vi "vision testing.vi"() -> ()   [LabVIEW 2013]
doc: "This VI demonstrates how to do target processing on a laptop computer. It uses the same MJPG VI as the dashboard, sets a few of the important camera properties that impact processing, and carries out the same processing steps as the RT example also included in this project."
uses:
  <vilib>/Rock Robotics/WPI/Camera/WPI_CameraImageSize.ctl
  <vilib>/vision/Image Controls.llb/IMAQ Image.ctl
  <vilib>/Rock Robotics/WPI/Camera/WPI_CameraWhite Balance Values.ctl
  <vilib>/Rock Robotics/WPI/Camera/WPI_CameraExposure Values.ctl
  <vilib>/Rock Robotics/WPI/Camera/WPI_CameraFrameRate.ctl
  <vilib>/vision/NI_Vision_Development_Module.lvlib
panel:
  out "final image":T1(plugin-control)
  in  "Pre-Process":bool
  out "mspi":u32=9
  in  "Numeric":i32=1
  out "y":dbl
  out "x":dbl
  out "Image Out":T1
  out "error out":errorcluster
  out "Number Found":i32
  in  "Camera Settings":T3={"FPS"=7, "Compression"=40, "Image Size"=enum."160x120"}
  in  "Camera IP Address":string="10.11.24.11"
  out "Original Image":T1(plugin-control)
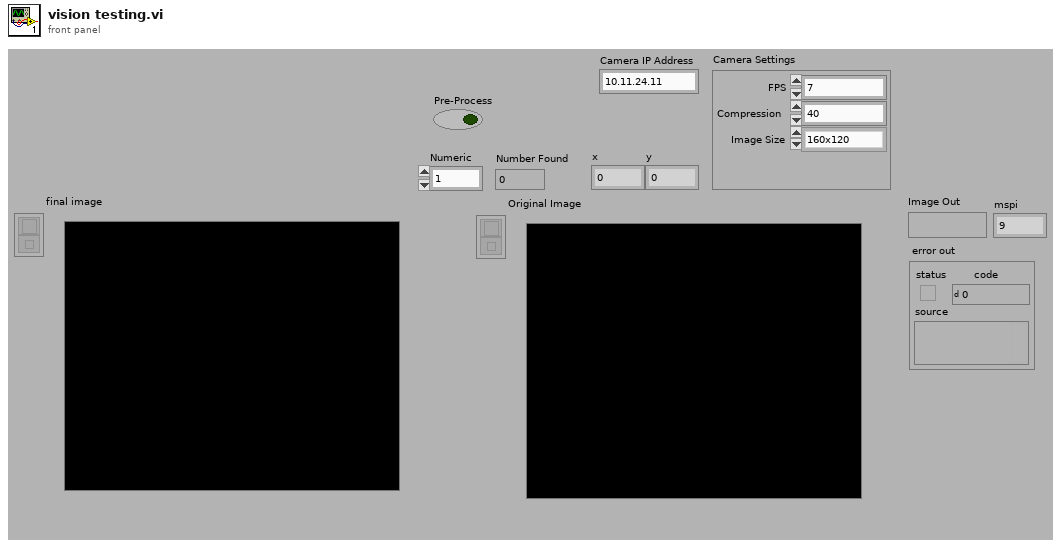
[diagram p1: front panel]
types:
  T1 = typedef "IMAQ Image.ctl" = refnum<image>
  T2 = typedef "WPI_CameraImageSize.ctl" = enum16{"640x480", "320x240", "160x120"}
  T3 = cluster{"FPS":i32, "Compression":i32, "Image Size":T2}
  T4 = typedef "Image Type" = u32
  T5 = typedef "WPI_CameraFrameRate.ctl" = u32
  T6 = typedef "WPI_CameraExposure Values.ctl" = enum16{"Auto", "Flicker-free 50 Hz", "Flicker-free 60 Hz", "Hold current"}
  T7 = typedef "WPI_CameraWhite Balance Values.ctl" = enum16{"Auto", "Fixed indoor", "Fixed outdoor 1", "Fixed outdoor 2", "Fixed fluorescent 1", "Fixed fluorescent 2", "Hold current"}
  T8 = typedef "WPI_CameraDevRef.ctl" = cluster{"Camera Address":string, "CameraStatus":errorcluster, "Acquire Image Notifier":refnum<notifier>}
  T9 = enum32{"AutoM", "Close", "Dilate", "Erode", "Gradient", "Gradient out", "Gradient in", "Hit miss", "Open", "PClose", "POpen", "Thick", "Thin"}
  T10 = cluster{"Brightness":sgl, "Contrast":sgl, "Gamma":sgl}
  T11 = cluster{"Measurement Parameter":i32, "Range Lower Value":dbl, "Range Upper Value":dbl, "Range":bool, "Measurement Type":bool}[]
  T12 = typedef "Particle Parameters" = i32
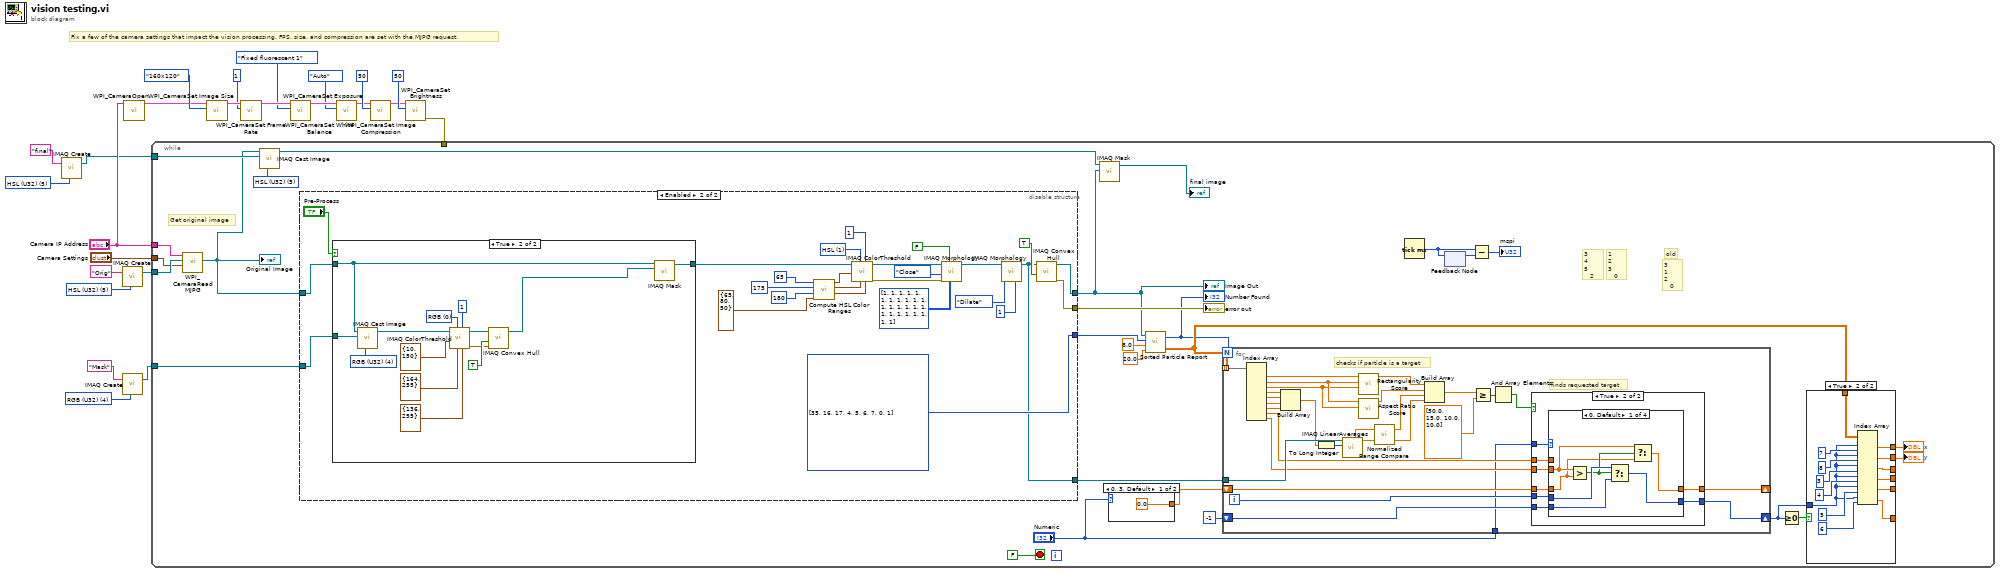
[diagram p0: block diagram]
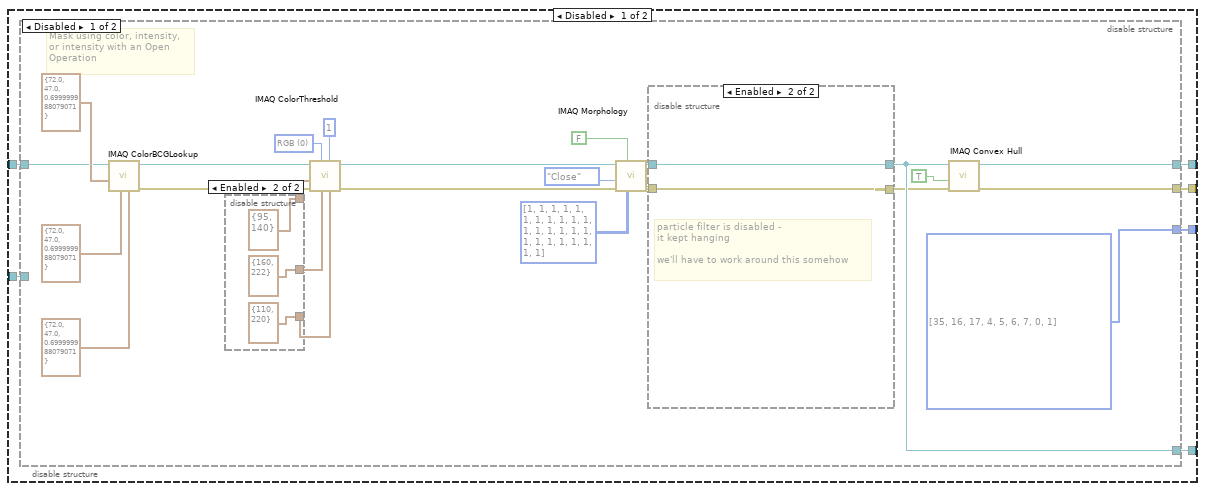
[diagram p2: hidden frame]
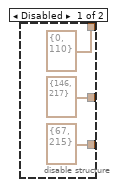
[diagram p3: hidden frame]
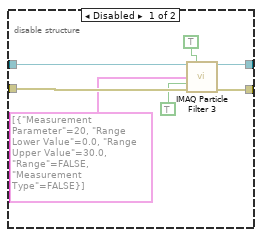
[diagram p4: hidden frame]
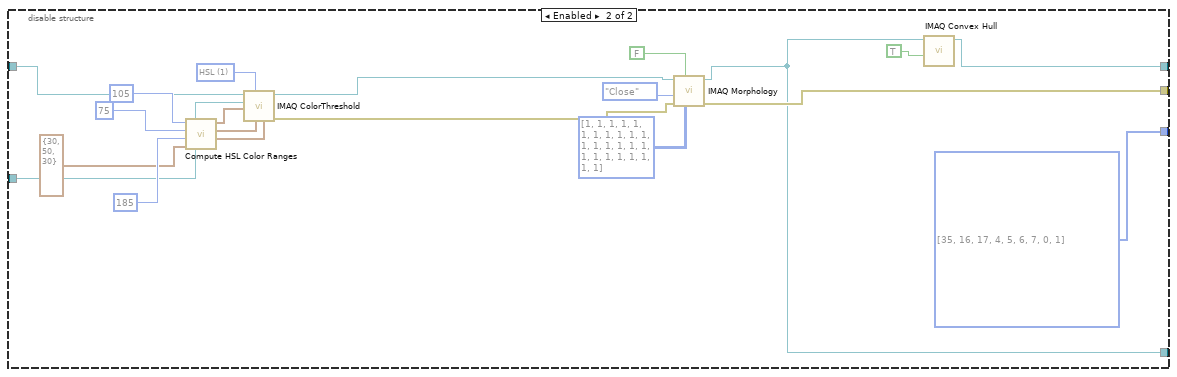
[diagram p5: hidden frame]
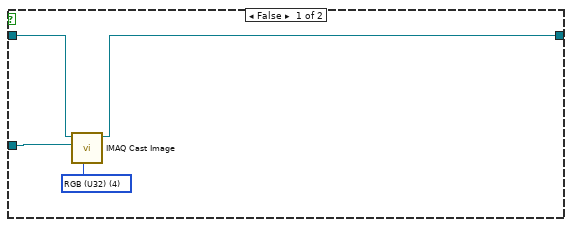
[diagram p6: hidden frame]
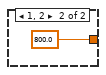
[diagram p7: hidden frame]
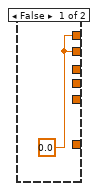
[diagram p8: hidden frame]
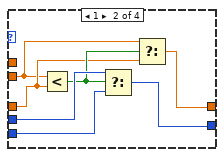
[diagram p10: hidden frame]
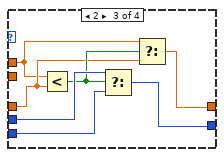
[diagram p11: hidden frame]
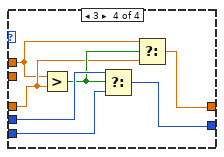
[diagram p12: hidden frame]
diagram:
  w3 = T4 5 items=["Grayscale (U8)", "Grayscale (I16)", "Grayscale (SGL)", "Complex (CSG)", "RGB (U32)", "HSL (U32)", "RGB (U64)", "Grayscale (U16)"] ("Image Type")
  w20 = T4 4 items=["Grayscale (U8)", "Grayscale (I16)", "Grayscale (SGL)", "Complex (CSG)", "RGB (U32)", "HSL (U32)", "RGB (U64)", "Grayscale (U16)"] ("Image Type")
  w23 = T4 5 items=["Grayscale (U8)", "Grayscale (I16)", "Grayscale (SGL)", "Complex (CSG)", "RGB (U32)", "HSL (U32)", "RGB (U64)", "Grayscale (U16)"] ("Image Type")
  # "Fix a few of the camera settings that impact the vision processing. FPS, size, and compression are set with the MJPG request."
  n1 = call "IMAQ Create"("Image Name"="final", "Image Type"=w3) -> ("New Image"=w1:T1)  [unwired: 2 in, 2 out]
  n2 = call "IMAQ Create"("Image Name"="Orig", "Image Type"=w23) -> ("New Image"=w22:T1)  [unwired: 2 in, 2 out]
  n3 = call "IMAQ Create"("Image Name"="Mask", "Image Type"=w20) -> ("New Image"=w19:T1)  [unwired: 2 in, 2 out]
  n4 = call <vilib>:"WPI_CameraOpen.vi"("Camera Address"="Camera IP Address") -> ("CameraDevRef"=w5:T8)  [unwired: 9 in, 1 out]
  n5 = call <vilib>:"WPI_CameraSet Image Size.vi"("Image Size"=WPI_CameraImageSize."160x120", "CameraDevRef"=w5) -> ("CameraDevRef Out"=w10:T8)  [unwired: 1 in, 8 out]
  n6 = call <vilib>:"WPI_CameraSet Frame Rate.vi"("Frame Rate (fps)"=T5 1, "CameraDevRef"=w10) -> ("CameraDevRef Out"=w12:T8)  [unwired: 1 in, 8 out]
  n7 = call <vilib>:"WPI_CameraSet White Balance.vi"("White Balance"=WPI_CameraWhite_Balance_Values."Fixed fluorescent 1", "CameraDevRef"=w12) -> ("CameraDevRef Out"=w11:T8)  [unwired: 1 in, 8 out]
  n8 = call <vilib>:"WPI_CameraSet Exposure.vi"("Exposure"=WPI_CameraExposure_Values."Auto", "CameraDevRef"=w11) -> ("CameraDevRef Out"=w14:T8)  [unwired: 1 in, 8 out]
  n9 = call <vilib>:"WPI_CameraSet Image Compression.vi"("Compression"=50, "CameraDevRef"=w14) -> ("CameraDevRef Out"=w13:T8)  [unwired: 1 in, 8 out]
  n10 = call <vilib>:"WPI_CameraSet Brightness.vi"("Brightness"=50, "CameraDevRef"=w13) -> ("error out"=w4:errorcluster)  [unwired: 1 in, 8 out]
  n11 = while {
    tunnel: w22 -> [w51]
    tunnel: w19 -> [w36]
    tunnel: "Camera IP Address" -> [w50]
    tunnel: "Camera Settings" -> [w49]
    tunnel: w4 -> [_]
    tunnel: w1 -> [w29]
    stop <- FALSE stop-if-true
    w30 = T4 5 items=["Grayscale (U8)", "Grayscale (I16)", "Grayscale (SGL)", "Complex (CSG)", "RGB (U32)", "HSL (U32)", "RGB (U64)"] ("Image Type")
    # "old"
    # "1   \n2     3\n   0"
    # "3   \n1     2\n   0"
    # "3   \n4     5\n   2"
    # "Get original image"
    n12 = call <vilib>:"WPI_CameraRead MJPG.vi"("Camera Settings"=w49, "Image"=w51, "address"=w50) -> ("Image Out"=w25:T1)  [unwired: 6 in, 2 out]
    "Original Image" <- w25
    n13 = call "IMAQ Cast Image"("Image Type"=w30, "Image Dst"=w29, "Image Src"=w25) -> ("Image Dst Out"=w28:T1)  [unwired: 7 in, 1 out]
    n14 = disable-structure shown="Enabled" {
      disable-tunnel: [w58 w143] -> w43
      disable-tunnel: [w57 w122] -> w40
      disable-tunnel: [w56 w120] -> w38
      disable-tunnel: w36 -> [w55 w141]
      disable-tunnel: w25 -> [w54 w140]
      disable-tunnel: [w53 w123] -> w26
      frame Disabled {
        n15 = disable-structure shown="Disabled" {
          disable-tunnel: [w82 w107] -> w58
          disable-tunnel: [w81 w98] -> w53
          disable-tunnel: [w80 w101] -> w57
          disable-tunnel: [w79 w99] -> w56
          disable-tunnel: w54 -> [w59 w109]
          disable-tunnel: w55 -> [_ w108]
          frame Disabled {
            w82 = T12[] [35, 16, 17, 4, 5, 6, 7, 0, 1] items=["Center of Mass X", "Center of Mass Y", "First Pixel X", "First Pixel Y", "Bounding Rect Left", "Bounding Rect Top", "Bounding Rect Right", "Bounding Rect Bottom", "Max Feret Diameter Start X", "Max Feret Diameter Start Y", "Max Feret Diameter End X", "Max Feret Diameter End Y", "Max Horiz. Segment Length Left", "Max Horiz. Segment Length Right", "Max Horiz. Segment Length Row", "-", "Bounding Rect Width", "Bounding Rect Height", "Bounding Rect Diagonal", "Perimeter", "Convex Hull Perimeter", "Holes' Perimeter", "Max Feret Diameter", "Equivalent Ellipse Major Axis", "Equivalent Ellipse Minor Axis", "Equivalent Ellipse Minor Axis (Feret)", "Equivalent Rect Long Side", "Equivalent Rect Short Side", "Equivalent Rect Diagonal", "Equivalent Rect Short Side (Feret)", "Average Horiz. Segment Length", "Average Vert. Segment Length", "Hydraulic Radius", "Waddel Disk Diameter", "-", "Area", "Holes' Area", "Particle & Holes' Area", "Convex Hull Area", "Image Area", "-", "Number of Holes", "Number of Horiz. Segments", "Number of Vert. Segments", "-", "Orientation", "Max Feret Diameter Orientation", "-", "% Area/Image Area", "% Area/(Particle & Holes' Area)", "Ratio of Equivalent Ellipse Axes", "Ratio of Equivalent Rect Sides", "-", "Elongation Factor", "Compactness Factor", "Heywood Circularity Factor", "Type Factor", "-", "Sum X", "Sum Y", "Sum XX", "Sum XY", "Sum YY", "Sum XXX", "Sum XXY", "Sum XYY", "Sum YYY", "-", "Moment of Inertia XX", "Moment of Inertia XY", "Moment of Inertia YY", "Moment of Inertia XXX", "Moment of Inertia XXY", "Moment of Inertia XYY", "Moment of Inertia YYY", "Norm. Moment of Inertia XX", "Norm. Moment of Inertia XY", "Norm. Moment of Inertia YY", "Norm. Moment of Inertia XXX", "Norm. Moment of Inertia XXY", "Norm. Moment of Inertia XYY", "Norm. Moment of Inertia YYY", "Hu Moment 1", "Hu Moment 2", "Hu Moment 3", "Hu Moment 4", "Hu Moment 5", "Hu Moment 6", "Hu Moment 7"] ("Requested Particle Measurements")
            w66 = u16 0 items=["RGB", "HSL", "HSV", "HSI"] ("Color Mode")
            # "Mask using color, intensity,\nor intensity with an Open\nOperation"
            n16 = call "IMAQ ColorBCGLookup"("Blue BCG Values"=T10 {"Brightness"=72.0, "Contrast"=47.0, "Gamma"=0.7}, "Green BCG Values"=T10 {"Brightness"=72.0, "Contrast"=47.0, "Gamma"=0.7}, "Red BCG Values"=T10 {"Brightness"=72.0, "Contrast"=47.0, "Gamma"=0.7}, "Image Src"=w59) -> ("error out"=w61:errorcluster, "Image Dst Out"=w60:T1)  [unwired: 3 in, 3 out]
            n17 = disable-structure shown="Enabled" {
              disable-tunnel: [cluster{"Lower value":i32, "Upper value":i32} {"Lower value"=0, "Upper value"=110} ("Red or Hue Range") cluster{"Lower value":i32, "Upper value":i32} {"Lower value"=95, "Upper value"=140} ("Red or Hue Range")] -> w67
              disable-tunnel: [cluster{"Lower value":i32, "Upper value":i32} {"Lower value"=146, "Upper value"=217} ("Green or Sat Range") cluster{"Lower value":i32, "Upper value":i32} {"Lower value"=160, "Upper value"=222} ("Green or Sat Range")] -> w68
              disable-tunnel: [cluster{"Lower value":i32, "Upper value":i32} {"Lower value"=67, "Upper value"=215} ("Blue or Luma or Val or Inten Range") cluster{"Lower value":i32, "Upper value":i32} {"Lower value"=110, "Upper value"=220} ("Blue or Luma or Val or Inten Range")] -> w69
              frame Disabled {
              }
              frame Enabled {
              }
            }
            n18 = call "IMAQ ColorThreshold"("Blue or Luma or Val or Inten Range"=w69, "Replace Value"=1, "Green or Sat Range"=w68, "Color Mode"=w66, "error in (no error)"=w61, "Red or Hue Range"=w67, "Image Src"=w60) -> ("error out"=w70:errorcluster, "Image Dst Out"=w74:T1)  [unwired: 1 in, 2 out]
            n19 = call "IMAQ Morphology"("Structuring Element"=i32[][] [[1, 1, 1, 1, 1], [1, 1, 1, 1, 1], [1, 1, 1, 1, 1], [1, 1, 1, 1, 1], [1, 1, 1, 1, 1]], "Square/Hexa (Square)"=FALSE, "error in (no error)"=w70, "Operation"=T9."Close", "Image Src"=w74) -> ("error out"=w75:errorcluster, "Image Dst Out"=w77:T1)  [unwired: 2 in, 3 out]
            n20 = disable-structure shown="Enabled" {
              disable-tunnel: w75 -> [w95 w96]
              disable-tunnel: [w92 w96] -> w76
              disable-tunnel: w77 -> [w91 w97]
              disable-tunnel: [w89 w97] -> w79
              frame Disabled {
                n21 = call "IMAQ Particle Filter 3"("Image Src"=w91, "Connectivity 4/8 (8)"=TRUE, "Selection Values"=T11 [{"Measurement Parameter"=20, "Range Lower Value"=0.0, "Range Upper Value"=30.0, "Range"=FALSE, "Measurement Type"=FALSE}], "Keep/Remove Particles (F)"=TRUE ("Keep/Remove Particles"), "error in (no error)"=w95) -> ("Image Dst Out"=w89:T1, "error out"=w92:errorcluster)  [unwired: 4 in, 5 out]
              }
              frame Enabled {
                # "particle filter is disabled - \nit kept hanging\n\nwe'll have to work around this somehow"
              }
            }
            n22 = call "IMAQ Convex Hull"("error in (no error)"=w76, "Connectivity 4/8 (8)"=TRUE, "Image Src"=w79) -> ("error out"=w80:errorcluster, "Image Dst Out"=w81:T1)  [unwired: 1 in, 6 out]
          }
          frame Enabled {
            w107 = T12[] [35, 16, 17, 4, 5, 6, 7, 0, 1] items=["Center of Mass X", "Center of Mass Y", "First Pixel X", "First Pixel Y", "Bounding Rect Left", "Bounding Rect Top", "Bounding Rect Right", "Bounding Rect Bottom", "Max Feret Diameter Start X", "Max Feret Diameter Start Y", "Max Feret Diameter End X", "Max Feret Diameter End Y", "Max Horiz. Segment Length Left", "Max Horiz. Segment Length Right", "Max Horiz. Segment Length Row", "-", "Bounding Rect Width", "Bounding Rect Height", "Bounding Rect Diagonal", "Perimeter", "Convex Hull Perimeter", "Holes' Perimeter", "Max Feret Diameter", "Equivalent Ellipse Major Axis", "Equivalent Ellipse Minor Axis", "Equivalent Ellipse Minor Axis (Feret)", "Equivalent Rect Long Side", "Equivalent Rect Short Side", "Equivalent Rect Diagonal", "Equivalent Rect Short Side (Feret)", "Average Horiz. Segment Length", "Average Vert. Segment Length", "Hydraulic Radius", "Waddel Disk Diameter", "-", "Area", "Holes' Area", "Particle & Holes' Area", "Convex Hull Area", "Image Area", "-", "Number of Holes", "Number of Horiz. Segments", "Number of Vert. Segments", "-", "Orientation", "Max Feret Diameter Orientation", "-", "% Area/Image Area", "% Area/(Particle & Holes' Area)", "Ratio of Equivalent Ellipse Axes", "Ratio of Equivalent Rect Sides", "-", "Elongation Factor", "Compactness Factor", "Heywood Circularity Factor", "Type Factor", "-", "Sum X", "Sum Y", "Sum XX", "Sum XY", "Sum YY", "Sum XXX", "Sum XXY", "Sum XYY", "Sum YYY", "-", "Moment of Inertia XX", "Moment of Inertia XY", "Moment of Inertia YY", "Moment of Inertia XXX", "Moment of Inertia XXY", "Moment of Inertia XYY", "Moment of Inertia YYY", "Norm. Moment of Inertia XX", "Norm. Moment of Inertia XY", "Norm. Moment of Inertia YY", "Norm. Moment of Inertia XXX", "Norm. Moment of Inertia XXY", "Norm. Moment of Inertia XYY", "Norm. Moment of Inertia YYY", "Hu Moment 1", "Hu Moment 2", "Hu Moment 3", "Hu Moment 4", "Hu Moment 5", "Hu Moment 6", "Hu Moment 7"] ("Requested Particle Measurements")
            w110 = u16 1 items=["RGB", "HSL", "HSV", "HSI"] ("Color Mode")
            n23 = call "Compute HSL Color Ranges.vi"("Margins"=cluster{"Hue":i32, "Sat":i32, "Lum":i32} {"Hue"=30, "Sat"=50, "Lum"=30}, "Luminance"=185, "Saturation"=75, "Hue"=105) -> ("Lum Range"=w113:cluster{i32, i32}, "Sat Range"=w112:cluster{i32, i32}, "Hue Range"=w111:cluster{i32, i32})  [unwired: 5 in]
            n24 = call "IMAQ ColorThreshold"("Blue or Luma or Val or Inten Range"=w113, "Green or Sat Range"=w112, "Color Mode"=w110, "Red or Hue Range"=w111, "Image Dst"=w108, "Image Src"=w109) -> ("error out"=w104:errorcluster, "Image Dst Out"=w105:T1)  [unwired: 4 in]
            n25 = call "IMAQ Morphology"("Structuring Element"=i32[][] [[1, 1, 1, 1, 1], [1, 1, 1, 1, 1], [1, 1, 1, 1, 1], [1, 1, 1, 1, 1], [1, 1, 1, 1, 1]], "Square/Hexa (Square)"=FALSE, "error in (no error)"=w104, "Operation"=T9."Close", "Image Src"=w105) -> ("error out"=w101:errorcluster, "Image Dst Out"=w99:T1)  [unwired: 2 in, 3 out]
            n26 = call "IMAQ Convex Hull"("Connectivity 4/8 (8)"=TRUE, "Image Src"=w99) -> ("Image Dst Out"=w98:T1)  [unwired: 2 in, 7 out]
          }
        }
      }
      frame Enabled {
        w128 = u16 1 items=["RGB", "HSL", "HSV", "HSI"] ("Color Mode")
        w143 = T12[] [35, 16, 17, 4, 5, 6, 7, 0, 1] items=["Center of Mass X", "Center of Mass Y", "First Pixel X", "First Pixel Y", "Bounding Rect Left", "Bounding Rect Top", "Bounding Rect Right", "Bounding Rect Bottom", "Max Feret Diameter Start X", "Max Feret Diameter Start Y", "Max Feret Diameter End X", "Max Feret Diameter End Y", "Max Horiz. Segment Length Left", "Max Horiz. Segment Length Right", "Max Horiz. Segment Length Row", "-", "Bounding Rect Width", "Bounding Rect Height", "Bounding Rect Diagonal", "Perimeter", "Convex Hull Perimeter", "Holes' Perimeter", "Max Feret Diameter", "Equivalent Ellipse Major Axis", "Equivalent Ellipse Minor Axis", "Equivalent Ellipse Minor Axis (Feret)", "Equivalent Rect Long Side", "Equivalent Rect Short Side", "Equivalent Rect Diagonal", "Equivalent Rect Short Side (Feret)", "Average Horiz. Segment Length", "Average Vert. Segment Length", "Hydraulic Radius", "Waddel Disk Diameter", "-", "Area", "Holes' Area", "Particle & Holes' Area", "Convex Hull Area", "Image Area", "-", "Number of Holes", "Number of Horiz. Segments", "Number of Vert. Segments", "-", "Orientation", "Max Feret Diameter Orientation", "-", "% Area/Image Area", "% Area/(Particle & Holes' Area)", "Ratio of Equivalent Ellipse Axes", "Ratio of Equivalent Rect Sides", "-", "Elongation Factor", "Compactness Factor", "Heywood Circularity Factor", "Type Factor", "-", "Sum X", "Sum Y", "Sum XX", "Sum XY", "Sum YY", "Sum XXX", "Sum XXY", "Sum XYY", "Sum YYY", "-", "Moment of Inertia XX", "Moment of Inertia XY", "Moment of Inertia YY", "Moment of Inertia XXX", "Moment of Inertia XXY", "Moment of Inertia XYY", "Moment of Inertia YYY", "Norm. Moment of Inertia XX", "Norm. Moment of Inertia XY", "Norm. Moment of Inertia YY", "Norm. Moment of Inertia XXX", "Norm. Moment of Inertia XXY", "Norm. Moment of Inertia XYY", "Norm. Moment of Inertia YYY", "Hu Moment 1", "Hu Moment 2", "Hu Moment 3", "Hu Moment 4", "Hu Moment 5", "Hu Moment 6", "Hu Moment 7"] ("Requested Particle Measurements")
        n27 = case shown="True" "Pre-Process" {
          tunnel: [w144 w161] -> w127
          tunnel: w141 -> [w146 w153]
          tunnel: w140 -> [w145 w152]
          frame False {
            w147 = T4 4 items=["Grayscale (U8)", "Grayscale (I16)", "Grayscale (SGL)", "Complex (CSG)", "RGB (U32)", "HSL (U32)", "RGB (U64)"] ("Image Type")
            n28 = call "IMAQ Cast Image"("Image Type"=w147, "Image Dst"=w146, "Image Src"=w145) -> ("Image Dst Out"=w144:T1)  [unwired: 7 in, 1 out]
          }
          frame True {
            w158 = u16 0 items=["RGB", "HSL", "HSV", "HSI"] ("Color Mode")
            w160 = T4 4 items=["Grayscale (U8)", "Grayscale (I16)", "Grayscale (SGL)", "Complex (CSG)", "RGB (U32)", "HSL (U32)", "RGB (U64)"] ("Image Type")
            n29 = call "IMAQ Cast Image"("Image Type"=w160, "Image Dst"=w153, "Image Src"=w152) -> ("Image Dst Out"=w156:T1)  [unwired: 7 in, 1 out]
            n30 = call "IMAQ ColorThreshold"("Blue or Luma or Val or Inten Range"=cluster{"Lower value":i32, "Upper value":i32} {"Lower value"=136, "Upper value"=255}, "Replace Value"=1, "Green or Sat Range"=cluster{"Lower value":i32, "Upper value":i32} {"Lower value"=164, "Upper value"=255}, "Color Mode"=w158, "Red or Hue Range"=cluster{"Lower value":i32, "Upper value":i32} {"Lower value"=10, "Upper value"=150}, "Image Src"=w156) -> ("error out"=w154:errorcluster, "Image Dst Out"=w155:T1)  [unwired: 2 in, 2 out]
            n31 = call "IMAQ Convex Hull"("error in (no error)"=w154, "Connectivity 4/8 (8)"=TRUE, "Image Src"=w155) -> ("Image Dst Out"=w151:T1)  [unwired: 7 in, 1 out]
            n32 = call "IMAQ Mask"("Image Mask"=w151, "Image Src"=w152) -> ("Image Dst Out"=w161:T1)  [unwired: 3 in, 1 out]
          }
        }
        n33 = call "Compute HSL Color Ranges.vi"("Margins"=cluster{"Hue":i32, "Sat":i32, "Lum":i32} {"Hue"=65, "Sat"=80, "Lum"=50}, "Luminance"=180, "Saturation"=175, "Hue"=65) -> ("Lum Range"=w131:cluster{i32, i32}, "Sat Range"=w130:cluster{i32, i32}, "Hue Range"=w129:cluster{i32, i32})  [unwired: 5 in]
        n34 = call "IMAQ ColorThreshold"("Blue or Luma or Val or Inten Range"=w131, "Replace Value"=1, "Green or Sat Range"=w130, "Color Mode"=w128, "Red or Hue Range"=w129, "Image Src"=w127) -> ("error out"=w125:errorcluster, "Image Dst Out"=w126:T1)  [unwired: 4 in]
        n35 = call "IMAQ Morphology"("Structuring Element"=i32[][] [[1, 1, 1, 1, 1], [1, 1, 1, 1, 1], [1, 1, 1, 1, 1], [1, 1, 1, 1, 1], [1, 1, 1, 1, 1]], "Square/Hexa (Square)"=FALSE, "error in (no error)"=w125, "Operation"=T9."Close", "Image Src"=w126) -> ("Image Dst Out"=w119:T1)  [unwired: 2 in, 4 out]
        n36 = call "IMAQ Morphology"("Number of iterations (1)"=1, "Operation"=T9."Dilate", "Image Src"=w119) -> ("Image Dst Out"=w120:T1)  [unwired: 7 in, 1 out]
        n37 = call "IMAQ Convex Hull"("Connectivity 4/8 (8)"=TRUE, "Image Src"=w120) -> ("error out"=w122:errorcluster, "Image Dst Out"=w123:T1)  [unwired: 8 in]
      }
    }
    "error out" <- w40
    "Image Out" <- w26
    n38 = call "IMAQ Mask"("Image Mask"=w26, "Image Src"=w28) -> ("Image Dst Out"=→"final image":T1)  [unwired: 3 in, 1 out]
    n39 = case shown="0, 3, Default" "Numeric" {
      tunnel: [0.0 ("element") 800.0 ("element")] -> w35
      frame 0, 3, Default {
      }
      frame 1, 2 {
      }
    }
    n40 = call "Sorted Particle Report.vi"("Area Size Limit"=20.0, "Particle Count Limit"=8.0, "Pixel Measurements"=w43, "Image in"=w26) -> ("Sorted Data"=w46:dbl[][], "Particles"=w37:i32)
    "Number Found" <- w37
    n41 = for {
      N: w37 -> [_]
      tunnel: w38 -> [w207]
      tunnel: w46 -> [w206] mode=indexing
      shift-right: [w189] -> _
      shift-left: w35 -> [w192]
      shift-right: [w190] -> w47
      shift-left: -1 -> [w191]
      tunnel: "Numeric" -> [w179]
      i -> [w193]
      # "checks if particle is a target"
      # "finds requested target"
      n42 = Index Array(array=w206) -> (element #1=w188:dbl, element #2=w185:dbl, element #3=w184:dbl, element #4=w202:dbl, element #5=w201:dbl, element #6=w200:dbl, element #7=w199:dbl, element #8=w195:dbl, element #9=w196:dbl)  [unwired: 9 in]
      n43 = Build Array(w202, w201, w200, w199) -> (w198:dbl[])
      n44 = To Long Integer(number=w198) -> (32bit integer=w197:i32[])
      n45 = call "IMAQ LinearAverages"("Optional Rectangle"=w197, "Image Src"=w207) -> ("Y Axis Averages"=w180:sgl[], "X Axis Averages"=w181:sgl[])  [unwired: 2 in, 6 out]
      n46 = call "Rectangularity Score.vi"("Height"=w184, "Width"=w185, "Area"=w188) -> ("Score"=w187:dbl)  [unwired: 8 in]
      n47 = call "Aspect Ratio Score.vi"("Height"=w184, "Width"=w185) -> ("Score"=w186:dbl)  [unwired: 8 in, 1 out]
      n48 = call "Normalized Range Compare.vi"("Y Averages"=w180, "X Averages"=w181) -> ("Y Score"=w182:dbl, "X Score"=w183:dbl)
      n49 = Build Array(w187, w186, w183, w182) -> (w205:dbl[])
      n50 = Greater Or Equal?(x=w205, y=dbl[] [50.0, 15.0, 10.0, 10.0]) -> (x >= y?=w203:bool[])
      n51 = And Array Elements(Boolean array=w203) -> (logical AND=w194:bool)
      n52 = case shown="True" w194 {
        tunnel: w196 -> [_ w217]
        tunnel: w195 -> [_ w216]
        tunnel: w193 -> [_ w215]
        tunnel: w192 -> [w208 w214]
        tunnel: w191 -> [w209 w213]
        tunnel: [w209 w212] -> w190
        tunnel: [w208 w211] -> w189
        tunnel: w179 -> [_ w210]
        frame False {
        }
        frame True {
          n53 = case shown="0, Default" w210 {
            tunnel: w217 -> [w220 w225 _ _]
            tunnel: w216 -> [_ _ w232 w239]
            tunnel: w215 -> [w224 w231 w238 w245]
            tunnel: w214 -> [w219 w227 w234 w241]
            tunnel: w213 -> [w223 w230 w237 w244]
            tunnel: [w222 w229 w236 w243] -> w212
            tunnel: [w218 w226 w233 w240] -> w211
            frame 0, Default {
              n54 = Greater?(x=w220, y=w219) -> (0:w221:bool)
              n55 = Select(t=w224, s=w221, f=w223) -> (s? t:f=w222:i32)
              n56 = Select(t=w220, s=w221, f=w219) -> (s? t:f=w218:dbl)
            }
            frame 1 {
              n57 = Less?(x=w225, y=w227) -> (x < y?=w228:bool)
              n58 = Select(t=w231, s=w228, f=w230) -> (s? t:f=w229:i32)
              n59 = Select(t=w225, s=w228, f=w227) -> (s? t:f=w226:dbl)
            }
            frame 2 {
              n60 = Less?(x=w232, y=w234) -> (x < y?=w235:bool)
              n61 = Select(t=w238, s=w235, f=w237) -> (s? t:f=w236:i32)
              n62 = Select(t=w232, s=w235, f=w234) -> (s? t:f=w233:dbl)
            }
            frame 3 {
              n63 = Greater?(x=w239, y=w241) -> (0:w242:bool)
              n64 = Select(t=w245, s=w242, f=w244) -> (s? t:f=w243:i32)
              n65 = Select(t=w239, s=w242, f=w241) -> (s? t:f=w240:dbl)
            }
          }
        }
      }
    }
    n66 = Tick Count (ms)() -> (millisecond timer value=w33:u32)
    n67 = feedback #1() -> (w32:u32)  [unwired: 1 in]
    n68 = feedback-in #1(w33) -> ()
    n69 = Subtract(x=w33, y=w32) -> (x-y=→"mspi":u32)
    n70 = Greater Or Equal To 0?(x=w47) -> (x >= 0?=w48:bool)
    n71 = case shown="True" w48 {
      tunnel: [w164 w176] -> w41
      tunnel: [w164 w175] -> w42
      tunnel: w46 -> [_ w174]
      tunnel: w47 -> [_ w170]
      tunnel: [_ w168] -> _
      tunnel: [_ w167] -> _
      tunnel: [_ w166] -> _
      tunnel: [_ w165] -> _
      frame False {
        w164 = 0.0 ("Numeric")
      }
      frame True {
        n72 = Index Array(array=w174, index (row) #1=w170, index (col) #1=7, index (row) #2=w170, index (col) #2=8, index (row) #3=w170, index (col) #3=3 ("index (row)"), index (row) #4=w170, index (col) #4=4 ("index (row)"), index (row) #5=w170, index (col) #5=5 ("index (row)"), index (row) #6=w170, index (col) #6=6 ("index (row)")) -> (element #1=w176:dbl, element #2=w175:dbl, element #3=w168:dbl, element #4=w165:dbl, element #5=w166:dbl, element #6=w167:dbl)
      }
    }
    "x" <- w41
    "y" <- w42
  }
